vi "getClusterElement.vi"(8 "error in (no error)":errorcluster, 10 "Label.Text":string, 11 "reference":refnum<vi>) -> (0 "error out":errorcluster, 2 "Value":variant, 3 "reference 2":refnum<vi>)   [LabVIEW 2016]
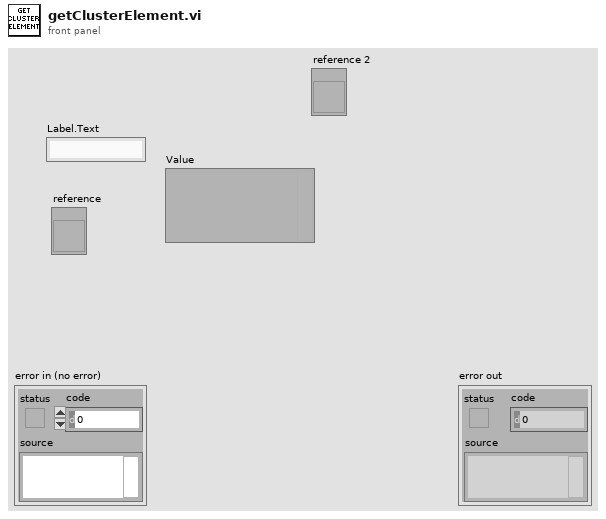
[diagram p1: front panel]
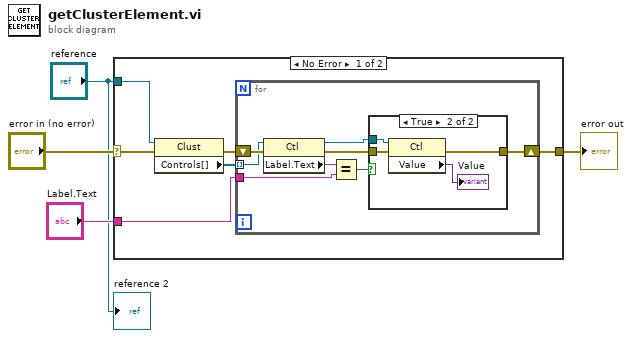
[diagram p0: block diagram]
diagram:
  n1 = case shown="No Error" "error in (no error)" {
    selector: "error in (no error)" -> [w8 w24]
    tunnel: [w7 w24] -> w3
    tunnel: "reference" -> [w6 _]
    tunnel: "Label.Text" -> [w5 _]
    frame No Error {
      n2 = property class="Clust"(reference=w6, error in=w8) -> (error out=w10:errorcluster, "Controls[]"=w9:refnum<vi>[])  [unwired: 1 out]
      n3 = for {
        shift-right: [w11] -> w7
        shift-left: w10 -> [w18]
        tunnel: w9 -> [w17] mode=indexing
        tunnel: w5 -> [w14]
        n4 = property class="Ctl"(reference=w17, error in=w18) -> (reference out=w12:refnum<vi>, error out=w16:errorcluster, "Label.Text"=w15:string)
        n5 = Equal?(x=w15, y=w14) -> (x = y?=w13:bool)
        n6 = case shown="True" w13 {
          tunnel: w16 -> [w19 w22]
          tunnel: w12 -> [_ w23]
          tunnel: [w19 w21] -> w11
          frame False {
          }
          frame True {
            n7 = property class="Ctl"(reference=w23, error in=w22) -> (error out=w21:errorcluster, "Value"=→"Value":variant)  [unwired: 1 out]
          }
        }
      }
    }
    frame Error {
    }
  }
  "error out" <- w3
  "reference 2" <- "reference"
